vi "get_graph_image.vi"(8 "error in":errorcluster, 10 "reference":refnum<vi>, 11 "Path":path) -> (0 "error out":errorcluster)   [LabVIEW 2016]
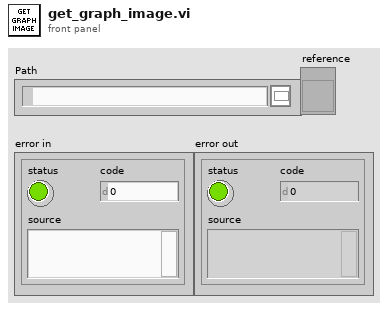
[diagram p1: front panel]
types:
  T1 = typedef "imagedata.ctl" = cluster{"image type":i32, "image depth":i32, "image":u8[], "mask":u8[], "colors":u32[], "Rectangle":cluster{"left":i16, "top":i16, "right":i16, "bottom":i16}}
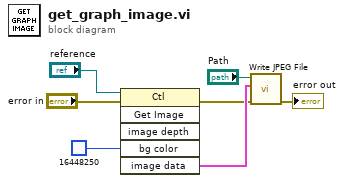
[diagram p0: block diagram]
diagram:
  n1 = invoke on="Invoke Node" class="Ctl" method="Get Image"(reference="reference", error in="error in", "bg color"=u32 16448250) -> (error out=w3:errorcluster, "image data"=w5:T1)  [unwired: 3 in, 4 out]
  n2 = call <vilib>:"Write JPEG File.vi"("error in (no error)"=w3, "image data"=w5, "path to JPEG file"="Path") -> ("error out"=→"error out":errorcluster)  [unwired: 7 in, 1 out]
